vi "Actor Core.vi"(8 "error in":errorcluster, 11 "Event Source in":refnum<class "Event Source.lvclass">) -> (0 "error out":errorcluster, 3 "Actor out":refnum<class "Actor.lvclass">)   [LabVIEW 2016, in "Event Source.lvlib" / "Event Source.lvclass"]
doc: "(<B>Filename</B>: Actor Framework.lvlib:Actor.lvclass:Actor Core.vi)\n\nReceives messages to the actor, reacts to them, and initiates any error handling that may shut the actor down.\n\nDescendant classes may override this VI to append parallel tasks for the actor to complete while it handles messages. Overrides use the Call Parent Method node."
uses:
  Event Source.lvclass
  <vilib>/ActorFramework/Actor/Actor.lvclass
  <vilib>/MGI/Monitored Actor/Monitored Actor/Monitored Actor/Monitored Actor.lvclass
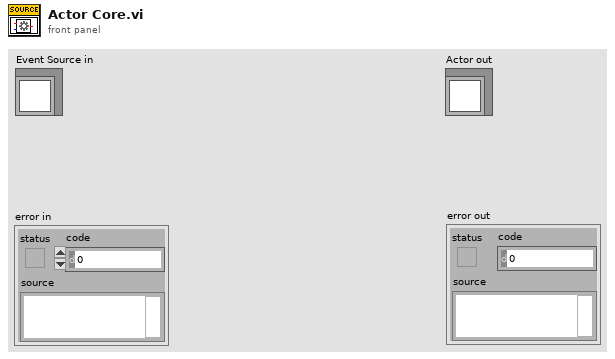
[diagram p1: front panel]
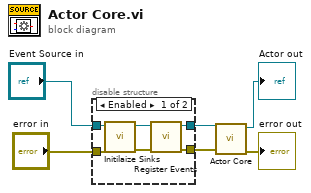
[diagram p0: block diagram]
diagram:
  n1 = disable-structure shown="Enabled" {
    disable-tunnel: "Event Source in" -> [w10 w14]
    disable-tunnel: [w9 w14] -> w3
    disable-tunnel: "error in" -> [w8 w13]
    disable-tunnel: [w7 w13] -> w1
    frame Enabled {
      n2 = call-dynamic "Initilaize Sinks.vi"("error in (no error)"=w8, "Event Source in"=w10) -> ("error out"=w12:errorcluster, "Event Source out"=w11:refnum<class "Event Source.lvclass">)  [unwired: 8 in]
      n3 = call-dynamic "Register Events.vi"("error in (no error)"=w12, "Event Source in"=w11) -> ("error out"=w7:errorcluster, "Event Source out"=w9:refnum<class "Event Source.lvclass">)  [unwired: 8 in]
    }
    frame Disabled {
    }
  }
  n4 = call-parent "Actor Core.vi"("error in"=w1, "Actor in"=w3) -> ("error out"=→"error out":errorcluster, "Actor out"=→"Actor out":refnum<class "Actor.lvclass">)  [unwired: 8 in]
